vi "Baseline Y at X.vi"(2 "min points to fit (100)":i32=100, 3 "X":dbl format="%.2f", 4 "baseline Y[]":dbl[](array[numeric]) format="%.2f", 5 "baseline X[]":dbl[](array[numeric]) format="%.2f") -> (1 "Y":dbl format="%.2f")   [LabVIEW 2012]
doc: "Calculates the Y value of the baseline at the given X (time). If there are at least 'min points to fit' baseline points in the baseline X and Y arrays, Y is calculated as a linear extrapolation of the baseline at X. Otherwise, Y is calculated as the average baseline Y value.\n\nUse the help window to read the descriptions of the individual controls for more information about this VI's inputs and outputs."
uses:
  <vilib>/Analysis/NI_AALPro.lvlib
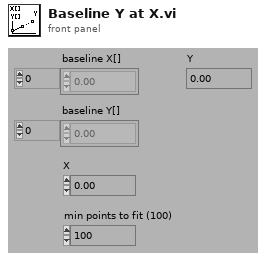
[diagram p1: front panel]
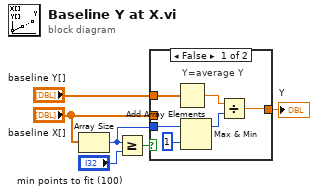
[diagram p0: block diagram]
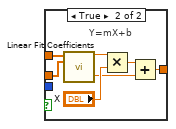
[diagram p2: hidden frame]
diagram:
  n1 = Array Size(array="baseline X[]") -> (size(s)=w2:i32)
  n2 = Greater Or Equal?(x=w2, y="min points to fit (100)") -> (x >= y?=w3:bool)
  n3 = case shown="False" w3 {
    tunnel: "baseline X[]" -> [_ w18]
    tunnel: "baseline Y[]" -> [w9 w19]
    tunnel: w2 -> [w8 _]
    tunnel: [w7 w13] -> w1
    frame False {
      # "Y=average Y"
      n4 = Add Array Elements(numeric array=w9) -> (sum=w10:dbl)
      n5 = Max & Min(x=w8, y=1) -> (max(x,y)=w12:i32)  [unwired: 1 out]
      n6 = Divide(x=w10, y=w12) -> (x/y=w7:dbl)
    }
    frame True {
      # "Y=mX+b"
      n7 = call <vilib>:"Linear Fit Coefficients.vi"("Y"=w19, "X"=w18) -> ("slope"=w16:dbl, "intercept"=w14:dbl)  [unwired: 11 in, 1 out]
      n8 = Multiply(x=w16, y="X") -> (x*y=w17:dbl)
      n9 = Add(x=w17, y=w14) -> (x+y=w13:dbl)
    }
  }
  "Y" <- w1
